vi "test_alignHorizontalCenterWithValidation.vi"(11 "Test Case In":refnum<class "RelativeAlignmentTests.lvclass">) -> (0 "error out":errorcluster, 3 "Test Case Out":refnum<class "RelativeAlignmentTests.lvclass">)   [LabVIEW 2023, in "RelativeAlignmentTests.lvclass"]
uses:
  RelativeAlignmentTests.lvclass
  <vilib>/Astemes/LUnit/Test Case.lvclass/Test Case.ctl
  <vilib>/Astemes/LUnit/Core/LUnit Test Case/Private/Append Fail Result.vi
  <vilib>/Astemes/LUnit/Core/LUnit Test Case/Private/Append Pass Result.vi
  <vilib>/Astemes/LUnit/Core/LUnit Test Case/Private/Run In UI.vi
  <vilib>/Utility/error.llb/Clear Errors.vi
  RelativeAlignmentTests.lvclass/RelativeAlignmentTests.ctl
  <vilib>/Astemes/LUnit/Test Case.lvclass
panel:
  in  "movingObject":string
  in  "anchor":dbl
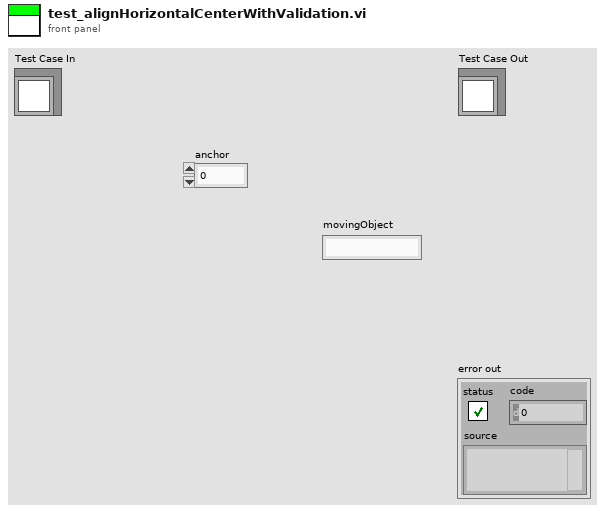
[diagram p1: front panel]
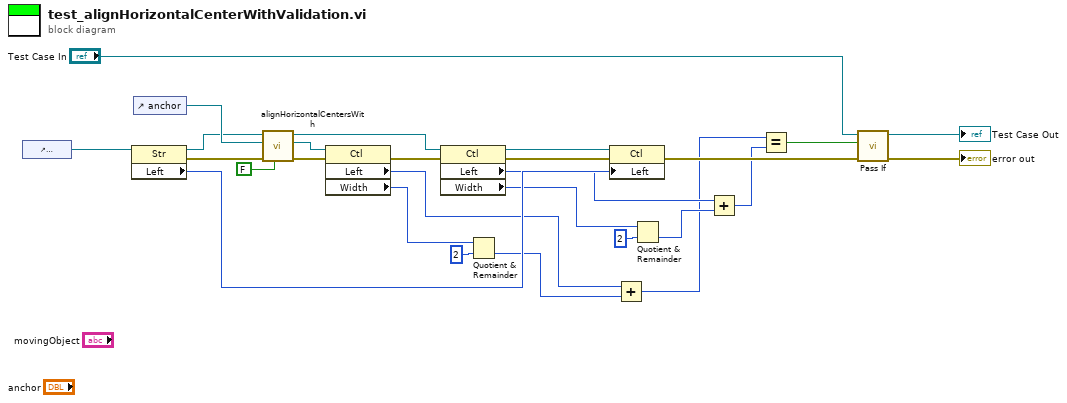
[diagram p0: block diagram]
diagram:
  n1 = control-ref of="movingObject"() -> (w18:refnum<vi>)
  n2 = property class="Str"(reference=w18) -> (reference out=w17:refnum<vi>, error out=w25:errorcluster, "Left"=w15:i32)  [unwired: 1 in]
  n3 = control-ref of="anchor"() -> (w26:refnum<vi>)
  n4 = call "alignHorizontalCentersWith.vi"("useControlBodyOnly"=FALSE, "error in (no error)"=w25, "anchorObject"=w26, "movingObject"=w17) -> ("error out"=w24:errorcluster, "anchorObject(dup)"=w22:refnum<vi>, "movingObject(dup)"=w21:refnum<vi>)  [unwired: 5 in]
  n5 = property class="Ctl"(reference=w22, error in=w24) -> (error out=w23:errorcluster, "Left"=w3:i32, "Width"=w4:u32)  [unwired: 1 out]
  n6 = property class="Ctl"(reference=w21, error in=w23) -> (reference out=w19:refnum<vi>, error out=w20:errorcluster, "Left"=w6:i32, "Width"=w8:u32)
  n7 = Quotient & Remainder(x=w4, y=u32 2) -> (floor(x/y)=w2:u32)  [unwired: 1 out]
  n8 = property class="Ctl"(reference=w19, error in=w20, "Left"=w15) -> (error out=w16:errorcluster)  [unwired: 1 out]
  n9 = Add(x=w3, y=w2) -> (x+y=w1:u32)
  n10 = Quotient & Remainder(x=w8, y=u32 2) -> (floor(x/y)=w7:u32)  [unwired: 1 out]
  n11 = Add(x=w6, y=w7) -> (x+y=w5:u32)
  n12 = Equal?(x=w1, y=w5) -> (x = y?=w14:bool)
  n13 = call <vilib>:"Pass If.vi"("error in (no error)"=w16, "Pass?"=w14, "LUnit Test Case In"="Test Case In") -> ("error out"=→"error out":errorcluster, "LUnit Test Case Out"=→"Test Case Out":refnum<class "RelativeAlignmentTests.lvclass">)  [unwired: 7 in]
